vi "LogVICall.vi"(8 "error in (no error)":errorcluster, 10 "StringEvent":string, 11 "EventLoggerData in":T1) -> (0 "error out":errorcluster, 3 "EventLoggerData out 2":T1)   [LabVIEW 2019, in "EventLogger.lvlib"]
uses:
  Cluster - EventLoggerData.ctl
  EventLogger.lvlib
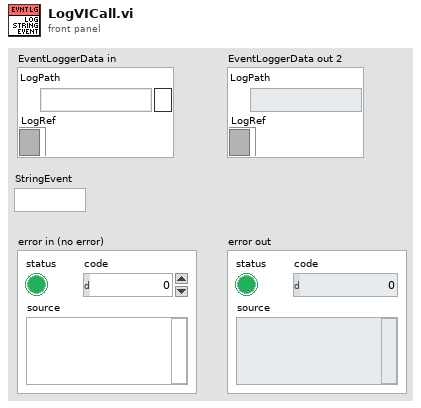
[diagram p1: front panel]
types:
  T1 = typedef "EventLogger.lvlib/Cluster - EventLoggerData.ctl" = cluster{"LogPath":path, "LogRef":refnum<file>}
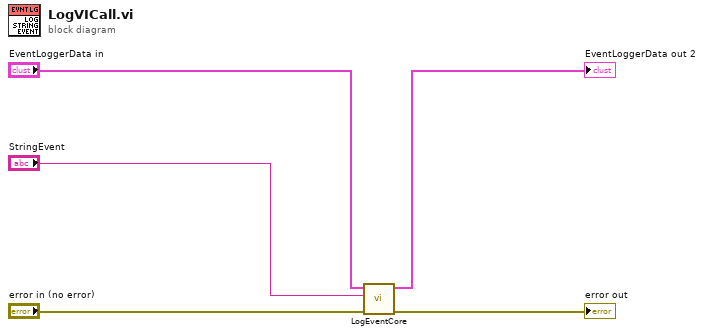
[diagram p0: block diagram]
diagram:
  n1 = call "LogEventCore.vi"("error in (no error)"="error in (no error)", "Event"="StringEvent", "EventLoggerData in in"="EventLoggerData in") -> ("error out"=→"error out":errorcluster, "EventLoggerData out"=→"EventLoggerData out 2":T1)  [unwired: 7 in]
